vi "ListboxSymbols-FG.vi"(7 "Actions":T1(ring), 8 "error in (no error)":errorcluster, 9 "Symbol Name":string, 10 "Tag":string, 11 "ListboxRef":refnum<vi>) -> (0 "error out":errorcluster, 1 "Symbol Index":i32, 2 "Item Tag out":string, 3 "ListboxRef out":refnum<vi>)   [LabVIEW 2018]
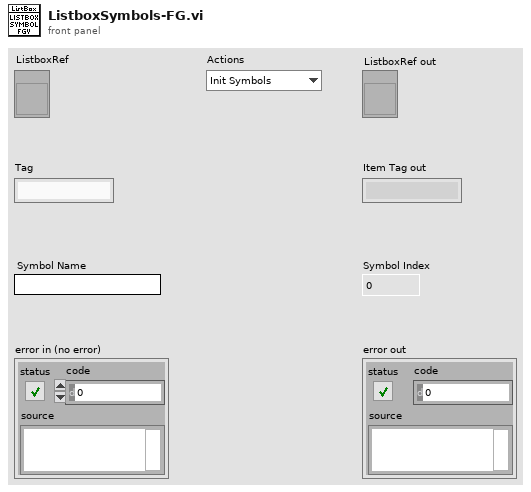
[diagram p1: front panel]
types:
  T1 = enum16{"Init Symbols", "Set Item Symbol", "Get Symbol Index"}
  T2 = typedef "imagedata.ctl" = cluster{"image type":i32, "image depth":i32, "image":u8[], "mask":u8[], "colors":u32[], "Rectangle":cluster{"left":i16, "top":i16, "right":i16, "bottom":i16}}
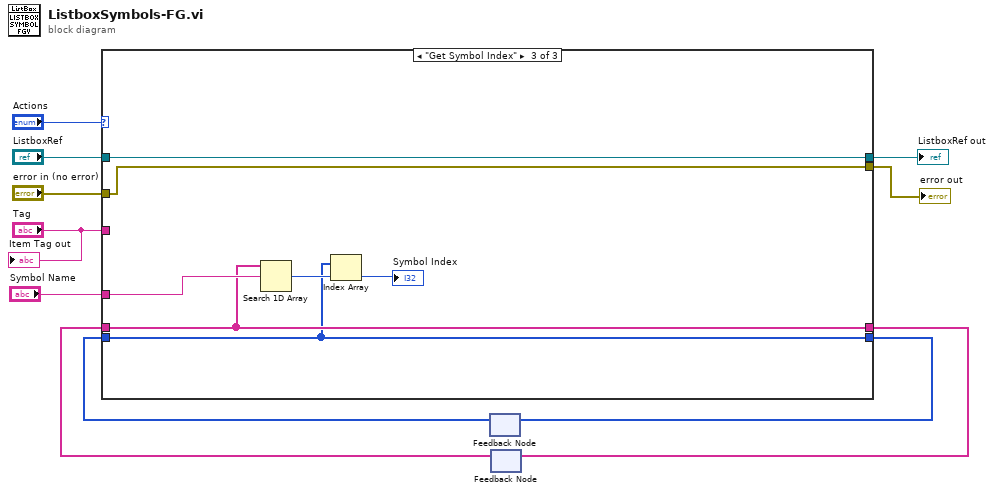
[diagram p0: block diagram]
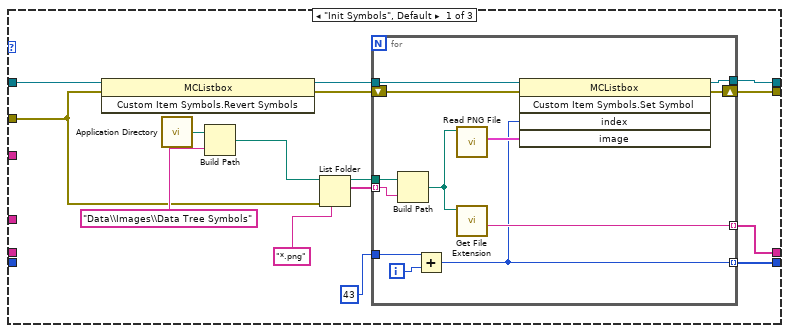
[diagram p2: hidden frame]
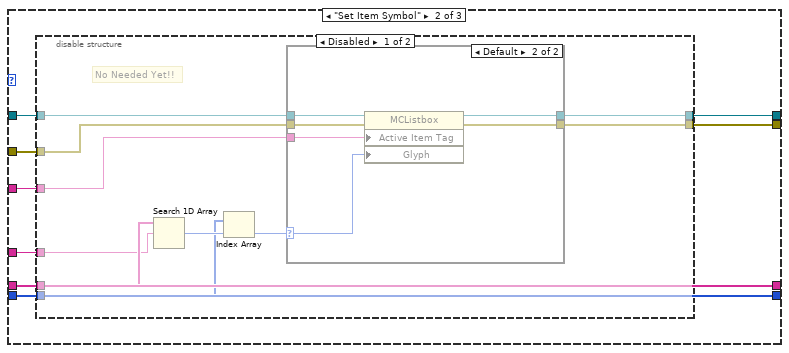
[diagram p3: hidden frame]
diagram:
  n1 = feedback #1() -> (w2:i32[])  [unwired: 1 in]
  n2 = feedback #2() -> (w3:string[])  [unwired: 1 in]
  n3 = case shown="\"Get Symbol Index\"" "Actions" {
    tunnel: "ListboxRef" -> [w26 w46 w73]
    tunnel: "error in (no error)" -> [w23 w45 w69]
    tunnel: [w15 w40 w68] -> w7
    tunnel: [w14 w41 w67] -> w8
    tunnel: [w13 w43 w73] -> w6
    tunnel: [w12 w42 w69] -> w5
    tunnel: "Tag" -> [_ w44 _]
    tunnel: w3 -> [_ w40 w68]
    tunnel: w2 -> [_ w41 w67]
    tunnel: "Symbol Name" -> [_ w39 w71]
    frame "Init Symbols", Default {
      n4 = invoke class="MCListbox" method="Custom Item Symbols.Revert Symbols"(reference=w26, error in=w23) -> (reference out=w20:refnum<vi>, error out=w19:errorcluster)  [unwired: 1 in, 1 out]
      n5 = call <vilib>:"Application Directory.vi"() -> ("Application Directory"=w25:path)
      n6 = Build Path(base path=w25, name or relative path="Data\\Images\\Data Tree Symbols") -> (appended path=w22:path)
      n7 = List Folder(path=w22, pattern="*.png", error in=w23) -> (path out=w18:path, filenames=w17:string[])  [unwired: 1 in, 2 out]
      n8 = for {
        tunnel: w20 -> [w37]
        shift-right: [w38] -> w12
        shift-left: w19 -> [w36]
        tunnel: [w35] -> w13
        tunnel: w18 -> [w34]
        tunnel: w17 -> [w33] mode=indexing
        tunnel: [w30] -> w15 mode=indexing
        tunnel: 43 -> [w28]
        tunnel: [w27] -> w14 mode=indexing
        i -> [w29]
        n9 = Build Path(base path=w34, name or relative path=w33) -> (appended path=w31:path)
        n10 = Add(x=w28, y=w29) -> (x+y=w27:i32)
        n11 = call <vilib>:"Read PNG File.vi"("path to PNG file"=w31) -> ("image data"=w32:T2)  [unwired: 8 in, 2 out]
        n12 = call <vilib>:"Get File Extension.vi"("file"=w31) -> ("filename without extension"=w30:string)  [unwired: 6 in, 4 out]
        n13 = invoke class="MCListbox" method="Custom Item Symbols.Set Symbol"(reference=w37, error in=w36, "index"=w27, "image"=w32) -> (reference out=w35:refnum<vi>, error out=w38:errorcluster)  [unwired: 1 in, 3 out]
      }
    }
    frame "Set Item Symbol" {
      n14 = disable-structure shown="Disabled" {
        disable-tunnel: w46 -> [w56 w66]
        disable-tunnel: w45 -> [w55 w65]
        disable-tunnel: w44 -> [w54 _]
        disable-tunnel: [w53 w66] -> w43
        disable-tunnel: [w52 w65] -> w42
        disable-tunnel: w41 -> [w49 _]
        disable-tunnel: w40 -> [w48 _]
        disable-tunnel: w39 -> [w47 _]
        frame Disabled {
          # "No Needed Yet!!"
          n15 = Search 1D Array(1D array=w48, element=w47) -> (index of element=w51:i32)  [unwired: 1 in]
          n16 = Index Array(array=w49, index=w51) -> (element=w50:i32)
          n17 = case shown="Default" w50 {
            selector: w50 -> [_ w59]
            tunnel: w56 -> [w58 w64]
            tunnel: w55 -> [w57 w63]
            tunnel: w54 -> [_ w62]
            tunnel: [w58 w61] -> w53
            tunnel: [w57 w60] -> w52
            frame -1 {
            }
            frame Default {
              n18 = property class="MCListbox"(reference=w64, error in=w63, "Active Item Tag"=w62, "Glyph"=w59) -> (reference out=w61:refnum<vi>, error out=w60:errorcluster)
            }
          }
        }
        frame Enabled {
        }
      }
    }
    frame "Get Symbol Index" {
      n19 = Search 1D Array(1D array=w68, element=w71) -> (index of element=w72:i32)  [unwired: 1 in]
      n20 = Index Array(array=w67, index=w72) -> (element=→"Symbol Index":i32)
    }
  }
  "ListboxRef out" <- w6
  "error out" <- w5
  n21 = feedback-in #1(w8) -> ()
  n22 = feedback-in #2(w7) -> ()
  "Item Tag out" <- "Tag"
